vi "newITaskClass.vi"(8 "error in (no error)":errorcluster, 10 "stopMechanismType":T1=enum."BooleanUE", 11 "classPath":path) -> (0 "error out":errorcluster, 3 "classPath(dup)":path)   [LabVIEW 2023]
uses:
  stopMechanismType.ctl
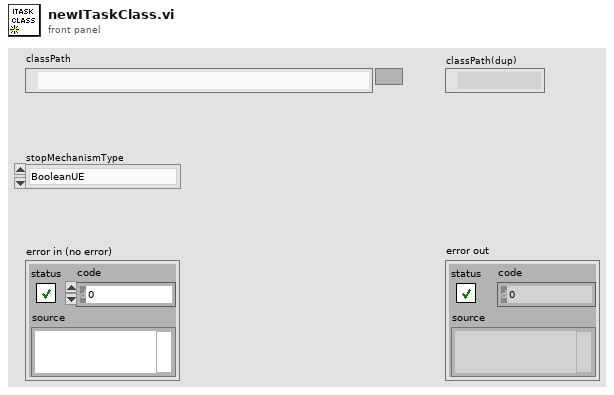
[diagram p1: front panel]
types:
  T1 = typedef "stopMechanismType.ctl" = enum16{"BooleanNotifier", "BooleanUE", "MsgUE", "MsgQueue"}
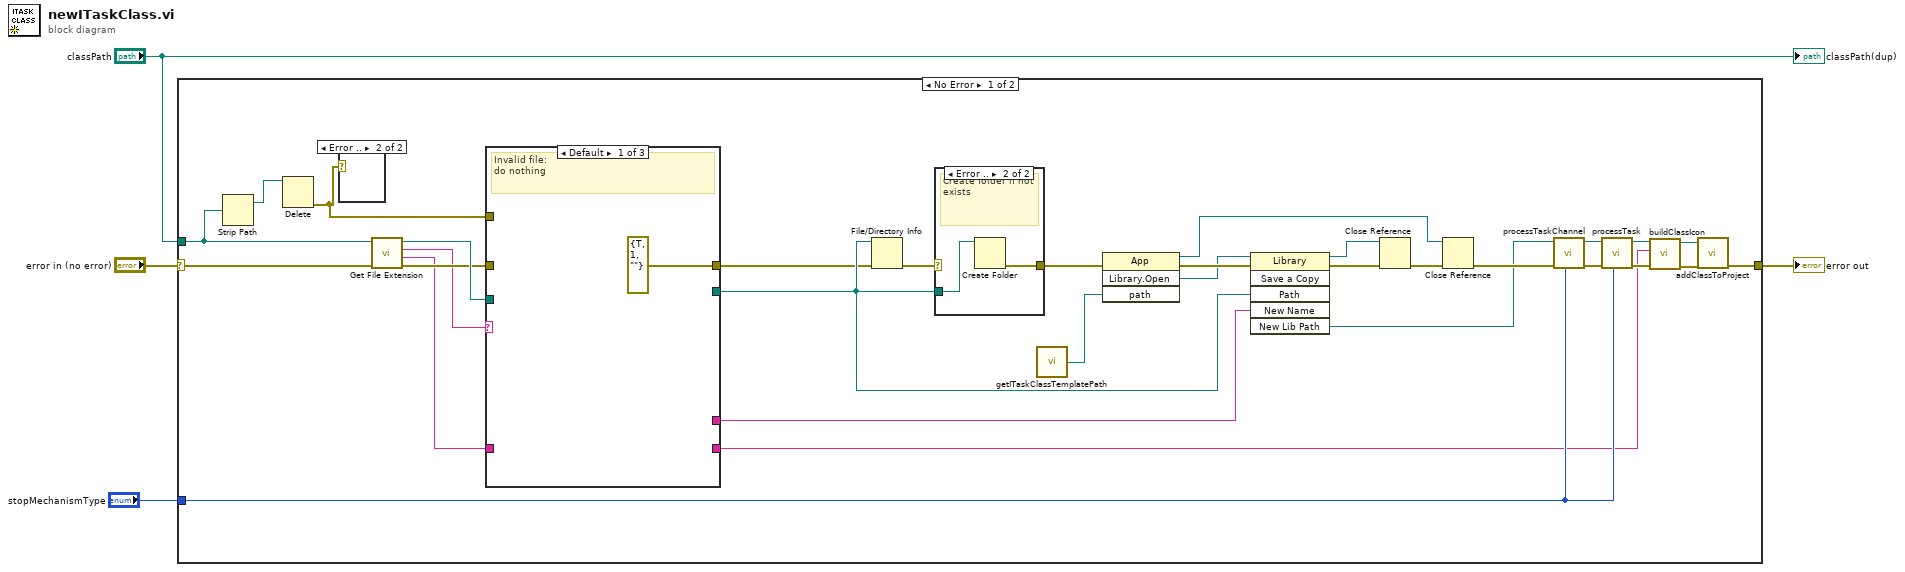
[diagram p0: block diagram]
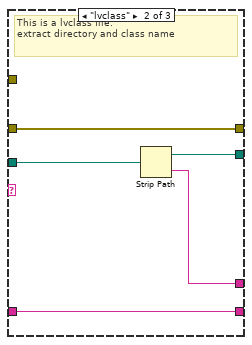
[diagram p4: hidden frame]
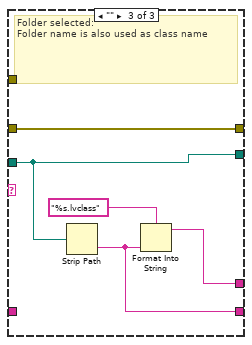
[diagram p5: hidden frame]
diagram:
  n1 = case shown="No Error" "error in (no error)" {
    selector: "error in (no error)" -> [w31 w50]
    tunnel: "classPath" -> [w16 _]
    tunnel: [w11 w50] -> w3
    tunnel: "stopMechanismType" -> [w10 _]
    frame No Error {
      n2 = Strip Path(path=w16) -> (stripped path=w15:path)  [unwired: 1 out]
      n3 = Delete(path (use dialog)=w15) -> (error out=w14:errorcluster)  [unwired: 4 in, 2 out]
      n4 = case shown="Error .." w14 {
        frame No Error {
        }
        frame Error {
        }
      }
      n5 = call <vilib>:"Get File Extension.vi"("error in (no error)"=w31, "file"=w16) -> ("error out"=w30:errorcluster, "filename without extension"=w24:string, "lowercase file extension"=w29:string, "dup file"=w35:path)  [unwired: 5 in, 1 out]
      n6 = case shown="Default" w29 {
        tunnel: w35 -> [_ w44 w47]
        tunnel: [_ w42 w48] -> w34
        tunnel: [_ w43 w47] -> w33
        tunnel: [errorcluster {"status"=TRUE, "code"=1, "source"=""} ("error in") w41 w46] -> w32
        tunnel: w30 -> [_ w41 w46]
        tunnel: [_ w40 w45] -> w5
        tunnel: w24 -> [_ w40 _]
        tunnel: w14 -> [_ _ _]
        frame Default {
          # "Invalid file:\ndo nothing"
        }
        frame "lvclass" {
          # "This is a lvclass file:\nextract directory and class name"
          n7 = Strip Path(path=w44) -> (stripped path=w43:path, name=w42:string)
        }
        frame "" {
          # "Folder selected:\nFolder name is also used as class name"
          n8 = Strip Path(path=w47) -> (name=w45:string)  [unwired: 1 out]
          n9 = Format Into String(format string="%s.lvclass", w45) -> (resulting string=w48:string)  [unwired: 2 in, 1 out]
        }
      }
      n10 = File/Directory Info(path=w33, error in=w32) -> (error out=w28:errorcluster)  [unwired: 6 out]
      n11 = case shown="Error .." w28 {
        selector: w28 -> [w36 _]
        tunnel: w33 -> [_ w38]
        tunnel: [w36 w37] -> w26
        frame No Error {
        }
        frame Error {
          # "Create folder if not exists"
          n12 = Create Folder(path (use dialog)=w38) -> (error out=w37:errorcluster)  [unwired: 2 in, 2 out]
        }
      }
      n13 = call "getITaskClassTemplatePath.vi"() -> ("ITaskClassPath"=w27:path)
      n14 = invoke class="App" method="Library.Open"(error in=w26, "path"=w27) -> (reference out=w25:refnum<vi>, error out=w23:errorcluster, "Open Library"=w22:refnum<vi>)  [unwired: 2 in, 1 out]
      n15 = invoke class="Library" method="Save a Copy"(reference=w22, error in=w23, "Path"=w33, "New Name"=w34) -> (reference out=w21:refnum<vi>, error out=w20:errorcluster, "New Lib Path"=w17:path)  [unwired: 2 in, 3 out]
      n16 = Close Reference(reference=w21, error in (no error)=w20) -> (error out=w19:errorcluster)
      n17 = Close Reference(reference=w25, error in (no error)=w19) -> (error out=w18:errorcluster)
      n18 = call "processTaskChannel.vi"("taskChannel"=w10, "error in (no error)"=w18, "targetClassPath"=w17) -> ("error out"=w13:errorcluster, "targetClassPath(dup)"=w12:path)  [unwired: 7 in]
      n19 = call "processTask.vi"("taskChannelType"=w10, "error in (no error)"=w13, "classPath"=w12) -> ("error out"=w9:errorcluster, "classPath(dup)"=w7:path)  [unwired: 7 in]
      n20 = call "buildClassIcon.vi"("error in (no error)"=w9, "className"=w5, "targetClassPath"=w7) -> ("error out"=w8:errorcluster, "targetClassPath(dup)"=w6:path)  [unwired: 7 in]
      n21 = call "addClassToProject.vi"("error in (no error)"=w8, "targetClassPath"=w6) -> ("error out"=w11:errorcluster)  [unwired: 8 in, 1 out]
    }
    frame Error {
    }
  }
  "error out" <- w3
  "classPath(dup)" <- "classPath"
